vi "Read Section Name.vi"(8 "error in (no error)":errorcluster, 11 "Pages in":refnum<class "Pages.lvclass">) -> (0 "error out":errorcluster, 2 "Section Name":string, 3 "Pages out":refnum<class "Pages.lvclass">)   [LabVIEW 2019, in "Pages.lvclass"]
uses:
  Pages.lvclass
  Pages.lvclass/Pages.ctl
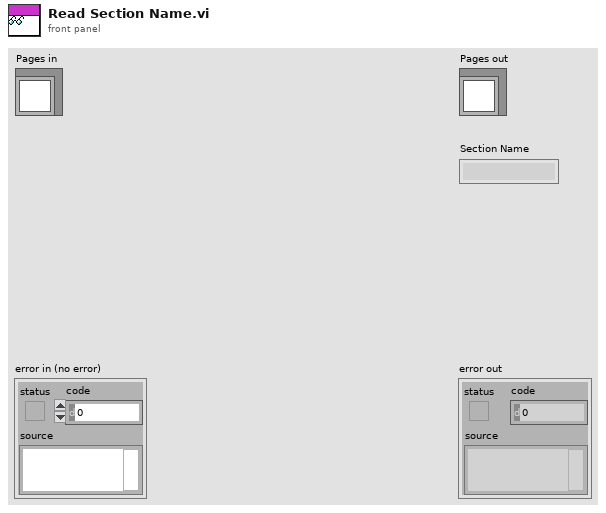
[diagram p1: front panel]
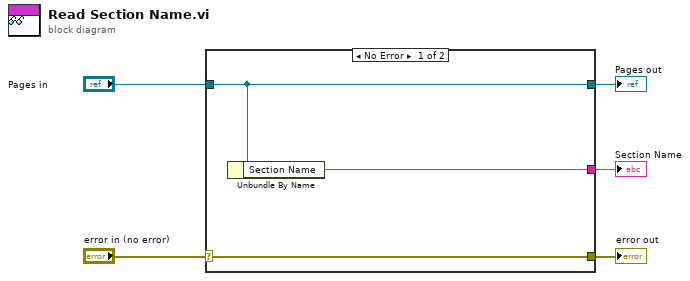
[diagram p0: block diagram]
diagram:
  n1 = case shown="No Error" "error in (no error)" {
    selector: "error in (no error)" -> [w8 w9]
    tunnel: [w8 w9] -> w4
    tunnel: [w7 w10] -> w2
    tunnel: "Pages in" -> [w7 w10]
    tunnel: [w6 _] -> w1
    frame No Error {
      n2 = Unbundle By Name(w7) -> ("Section Name"=w6:string)
    }
    frame Error {
    }
  }
  "error out" <- w4
  "Pages out" <- w2
  "Section Name" <- w1
